vi "Parse-attribute.vi"(8 "error in (no error)":errorcluster, 10 "String in":string, 11 "LaserOffDelay in":refnum<class "LaserOffDelay.lvclass">) -> (0 "error out":errorcluster, 1 "Valid attribute?":bool, 2 "Remaining string":string, 3 "LaserOffDelay out":refnum<class "LaserOffDelay.lvclass">)   [LabVIEW 2013, in "HardwareCharacterization.lvlib" / "LaserOffDelay.lvclass"]
uses:
  LaserOffDelay.lvclass
  Attributes.ctl
  Attribute-ID.ctl
  Attribute-XML.lvclass/Attribute-XML.ctl
  ID.lvclass/ID.ctl
  Time/Time.lvclass/Time.ctl
  Write Attribute.vi
  Write ID-attribute.vi
  Time/Write Time interval.vi
  Attribute-XML.lvclass
  ID.lvclass
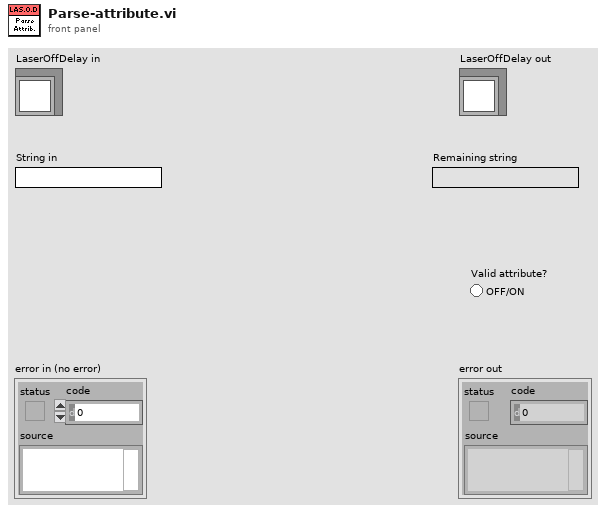
[diagram p1: front panel]
types:
  T1 = typedef "HardwareCharacterization.lvlib/ID.lvclass/Attribute-ID.ctl" = enum16{"FieldOffset", "TransformEnable", "Transform", "Units", "XYCalFactor", "EnableLaser", "JumpDelay", "MarkDelay", "PolyDelay", "LaserOnDelay", "LaserOffDelay", "JumpSpeed", "MarkSpeed", "LaserPowerDelay", "LaserEnableDelay", "LaserPower", "Offset"}
  T2 = typedef "HardwareCharacterization.lvlib/Attribute-XML.lvclass/Attributes.ctl" = enum16{"id"}
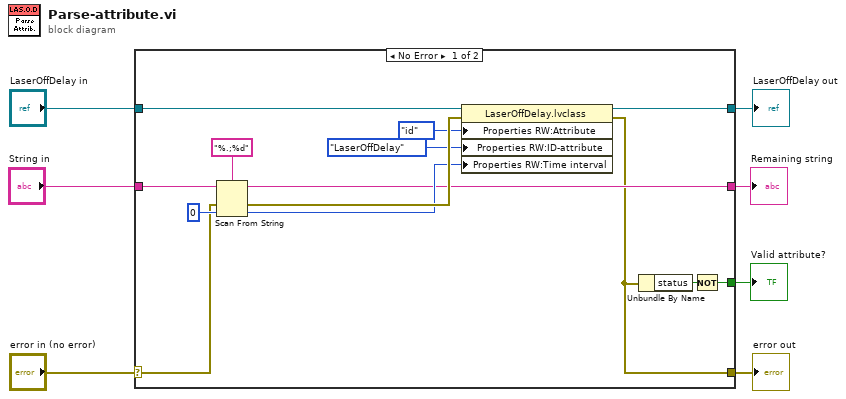
[diagram p0: block diagram]
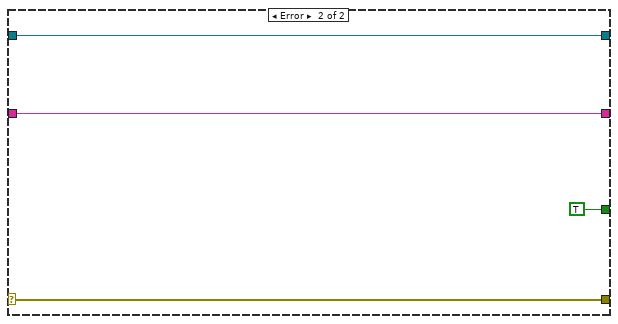
[diagram p2: hidden frame]
diagram:
  n1 = case shown="No Error" "error in (no error)" {
    selector: "error in (no error)" -> [w8 w25]
    tunnel: [w9 w25] -> w6
    tunnel: [w13 w24] -> w4
    tunnel: "LaserOffDelay in" -> [w14 w24]
    tunnel: "String in" -> [w12 w23]
    tunnel: [w11 w23] -> w2
    tunnel: [w10 TRUE] -> w1
    frame No Error {
      n2 = Scan From String(format string="%.;%d", input string=w12, error in=w8, default 1=i64 0 ("default value 2")) -> (remaining string=w11:string, error out=w19:errorcluster, output 1=w16:i64)  [unwired: 1 in, 1 out]
      n3 = property class="LaserOffDelay.lvclass"(reference=w14, error in=w19, "Properties RW:Attribute"=Attributes."id" ("Attribute"), "Properties RW:ID-attribute"=Attribute-ID."LaserOffDelay" ("ID-attribute"), "Properties RW:Time interval"=w16) -> (reference out=w13:refnum<class "LaserOffDelay.lvclass">, error out=w9:errorcluster)
      n4 = Unbundle By Name(w9) -> ("status"=w20:bool)
      n5 = Not(x=w20) -> (.not. x?=w10:bool)
    }
    frame Error {
    }
  }
  "error out" <- w6
  "LaserOffDelay out" <- w4
  "Valid attribute?" <- w1
  "Remaining string" <- w2
